vi "CVT2ParallelStaticTest.vi"() -> (3 "Unit Test Framework Results":T1)   [LabVIEW 2013, in "UnitTests.lvlib"]
uses:
  UnitTests.lvlib
  <vilib>/utf/common/utf_test_result_troll.ctl
  <vilib>/utf/common/utf_test_result.ctl
  <vilib>/utf/common/utf_test_result_failure.ctl
  <vilib>/utf/common/utf_test_comparison_operators.ctl
  <vilib>/utf/common/utf_vi_tag.ctl
  <vilib>/NI/Current Value Table/DataTypes/I32_Static Write.vi
  <vilib>/NI/Current Value Table/DataTypes/I32_Static Read.vi
  <vilib>/NI/Current Value Table/Type to Enum.vi
  <vilib>/NI/Current Value Table/DataTypes/I32_Type To Enum.vi
  <vilib>/NI/Current Value Table/FGVs/Tag Memory.vi
  <vilib>/NI/Current Value Table/Memory Block.vi
  <vilib>/NI/Current Value Table/DataTypes/I32_Memory Block.vi
  <vilib>/utf/NI_UnitTestFramework.lvlib
  <vilib>/NI/Current Value Table/Current Value Table.lvlib
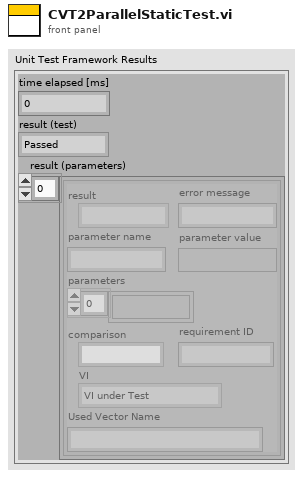
[diagram p1: front panel]
types:
  T1 = typedef "NI_UnitTestFramework.lvlib/utf_test_result_troll.ctl" = cluster{"time elapsed [ms]":u32, "result (test)":T2, "result (parameters)":T3[]}
  T2 = typedef "NI_UnitTestFramework.lvlib/utf_test_result.ctl" = enum16{"Passed", "Failed", "Error", "Skipped", "Not Processed"}
  T3 = typedef "NI_UnitTestFramework.lvlib/utf_test_result_failure.ctl" = cluster{"result":T2, "error message":string, "parameter name":string, "parameter value":variant, "parameters":variant[], "comparison":T4, "requirement ID":string, "VI":T5, "Used Vector Name":string}
  T4 = typedef "NI_UnitTestFramework.lvlib/utf_test_comparison_operators.ctl" = enum16{"=", "!=", ">", ">=", "<", "<=", "range", "symmetric tolerance", "asymmetric tolerance", "string contains", "string not contain", "array size", "string length", "array range", "by element", "array range (limit array)", "user-defined", "array contains", "array not contain", "vector length", "= (elm)", "!= (elm)", "= (case insensitive)", "!= (case insensitive)"}
  T5 = typedef "NI_UnitTestFramework.lvlib/utf_vi_tag.ctl" = enum16{"Setup VI", "VI under Test", "Teardown VI"}
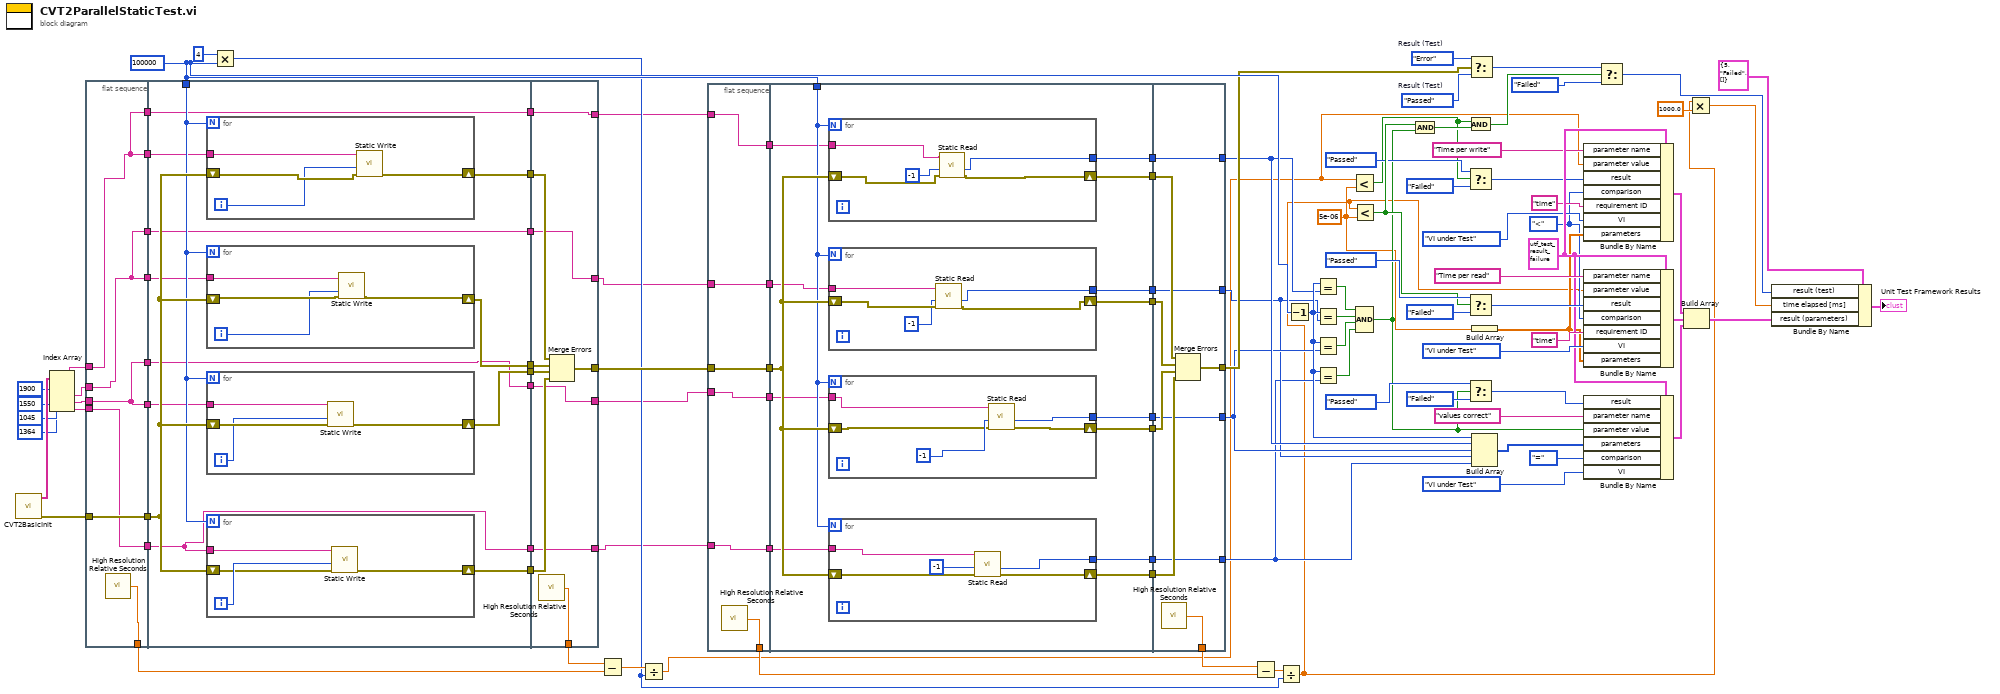
[diagram p0: block diagram]
diagram:
  w51 = T3 {"result"=enum."Passed", "error message"="", "parameter name"="", "parameter value"=variant, "parameters"=[], "comparison"=enum."=", "requirement ID"="", "VI"=enum."Setup VI", "Used Vector Name"=""} ("Unit Test Framework - result (parameters)")
  w31 = 5e-06 ("y")
  w42 = utf_test_comparison_operators."<" ("comparison")
  w87 = utf_test_result."Error"  # Result (Test)
  w86 = utf_test_result."Passed"  # Result (Test)
  w58 = 100000
  n1 = call "CVT2BasicInit.vi"() -> ("error out"=w66:errorcluster, "names"=w28:string[])  [unwired: 9 in, 1 out]
  n2 = Index Array(array=w28, index #1=1900 ("index"), index #2=1550 ("index"), index #3=1045 ("index"), index #4=1364 ("index")) -> (element #1=w17:string, element #2=w18:string, element #3=w20:string, element #4=w23:string)
  n3 = flat-sequence {
    tunnel: [w111] -> w105
    tunnel: [w112] -> w104
    tunnel: w66 -> [w112]
    tunnel: w23 -> [w110]
    tunnel: [w110] -> w22
    tunnel: [w107] -> w21
    tunnel: w20 -> [w107]
    tunnel: [w108] -> w19
    tunnel: w18 -> [w108]
    tunnel: w17 -> [w109]
    tunnel: [w109] -> w16
    tunnel: [w109] -> w12
    tunnel: [w108] -> w11
    tunnel: [w107] -> w4
    tunnel: w104 -> [w125]
    tunnel: [w124] -> w101
    tunnel: [w123] -> w100
    tunnel: [w122] -> w99
    tunnel: [w121] -> w98
    tunnel: w58 -> [w120]
    tunnel: w22 -> [w113]
    tunnel: w21 -> [w119]
    tunnel: w19 -> [w118]
    tunnel: w16 -> [w117]
    tunnel: [w116] -> w13
    tunnel: w12 -> [w116]
    tunnel: w11 -> [w115]
    tunnel: [w115] -> w10
    tunnel: [w114] -> w5
    tunnel: w4 -> [w114]
    tunnel: [w113] -> w3
    tunnel: [w146] -> w106
    tunnel: w101 -> [w151]
    tunnel: w100 -> [w150]
    tunnel: w99 -> [w149]
    tunnel: w98 -> [w148]
    tunnel: [w147] -> w92
    tunnel: [w145] -> w14
    tunnel: w13 -> [w145]
    tunnel: w10 -> [w144]
    tunnel: [w144] -> w9
    tunnel: [w143] -> w6
    tunnel: w5 -> [w143]
    tunnel: w3 -> [w142]
    tunnel: [w142] -> w2
    frame #0 {
      n4 = call <vilib>:"High Resolution Relative Seconds.vi"() -> ("relative seconds"=w111:dbl)
    }
    frame #1 {
      n5 = for {
        N: w120 -> [_]
        shift-right: [w139] -> w124
        shift-left: w125 -> [w140]
        tunnel: w117 -> [w141]
        i -> [w138]
        n6 = call-poly <vilib>:"Static Write.vi"("error in (no error)"=w140, "Value"=w138, "Tag Name"=w141) -> ("error out"=w139:errorcluster)  [unwired: 8 in]
      }
      n7 = for {
        N: w120 -> [_]
        shift-right: [w128] -> w123
        shift-left: w125 -> [w129]
        tunnel: w118 -> [w126]
        i -> [w127]
        n8 = call-poly <vilib>:"Static Write.vi"("error in (no error)"=w129, "Value"=w127, "Tag Name"=w126) -> ("error out"=w128:errorcluster)  [unwired: 8 in]
      }
      n9 = for {
        N: w120 -> [_]
        shift-right: [w137] -> w122
        shift-left: w125 -> [w136]
        tunnel: w119 -> [w134]
        i -> [w135]
        n10 = call-poly <vilib>:"Static Write.vi"("error in (no error)"=w136, "Value"=w135, "Tag Name"=w134) -> ("error out"=w137:errorcluster)  [unwired: 8 in]
      }
      n11 = for {
        N: w120 -> [_]
        shift-right: [w130] -> w121
        shift-left: w125 -> [w131]
        tunnel: w113 -> [w133]
        i -> [w132]
        n12 = call-poly <vilib>:"Static Write.vi"("error in (no error)"=w131, "Value"=w132, "Tag Name"=w133) -> ("error out"=w130:errorcluster)  [unwired: 8 in]
      }
    }
    frame #2 {
      n13 = call <vilib>:"High Resolution Relative Seconds.vi"() -> ("relative seconds"=w146:dbl)
      n14 = Merge Errors(w151, w150, w149, w148) -> (w147:errorcluster)
    }
  }
  n15 = Multiply(x=4, y=w58) -> (x*y=w54:i32)
  n16 = Subtract(x=w106, y=w105) -> (x-y=w56:dbl)
  n17 = Divide(x=w56, y=w54) -> (x/y=w29:dbl)
  n18 = flat-sequence {
    tunnel: [w156] -> w103
    tunnel: [w157] -> w97
    tunnel: w92 -> [w157]
    tunnel: [w155] -> w15
    tunnel: w14 -> [w155]
    tunnel: w9 -> [w154]
    tunnel: [w154] -> w8
    tunnel: [w153] -> w7
    tunnel: w6 -> [w153]
    tunnel: w2 -> [w152]
    tunnel: [w152] -> w1
    tunnel: w97 -> [w171]
    tunnel: [w170] -> w96
    tunnel: [w169] -> w95
    tunnel: [w168] -> w94
    tunnel: [w167] -> w93
    tunnel: w58 -> [w166]
    tunnel: [w165] -> w91
    tunnel: [w164] -> w65
    tunnel: [w163] -> w64
    tunnel: [w162] -> w63
    tunnel: w15 -> [w161]
    tunnel: w8 -> [w160]
    tunnel: w7 -> [w159]
    tunnel: w1 -> [w158]
    tunnel: [w201] -> w102
    tunnel: w96 -> [w195]
    tunnel: w95 -> [w194]
    tunnel: w94 -> [w193]
    tunnel: w93 -> [w192]
    tunnel: w91 -> [w199]
    tunnel: w65 -> [w197]
    tunnel: w64 -> [w198]
    tunnel: w63 -> [w200]
    tunnel: [w196] -> w53
    tunnel: [w195] -> w35
    tunnel: [w194] -> w33
    tunnel: [w193] -> w34
    tunnel: [w192] -> w32
    frame #0 {
      n19 = call <vilib>:"High Resolution Relative Seconds.vi"() -> ("relative seconds"=w156:dbl)
    }
    frame #1 {
      n20 = for {
        N: w166 -> [_]
        shift-right: [w191] -> w163
        shift-left: w171 -> [w187]
        tunnel: [w190] -> w170
        tunnel: w161 -> [w189]
        n21 = call-poly <vilib>:"Static Read.vi"("error in (no error)"=w187, "Default"=-1, "Tag Name"=w189) -> ("error out"=w191:errorcluster, "Value"=w190:i32)  [unwired: 7 in]
      }
      n22 = for {
        N: w166 -> [_]
        shift-right: [w172] -> w164
        shift-left: w171 -> [w175]
        tunnel: [w173] -> w169
        tunnel: w160 -> [w176]
        n23 = call-poly <vilib>:"Static Read.vi"("error in (no error)"=w175, "Default"=-1, "Tag Name"=w176) -> ("error out"=w172:errorcluster, "Value"=w173:i32)  [unwired: 7 in]
      }
      n24 = for {
        N: w166 -> [_]
        shift-right: [w183] -> w165
        shift-left: w171 -> [w184]
        tunnel: [w186] -> w168
        tunnel: w159 -> [w182]
        n25 = call-poly <vilib>:"Static Read.vi"("error in (no error)"=w184, "Default"=-1, "Tag Name"=w182) -> ("error out"=w183:errorcluster, "Value"=w186:i32)  [unwired: 7 in]
      }
      n26 = for {
        N: w166 -> [_]
        shift-right: [w177] -> w162
        shift-left: w171 -> [w181]
        tunnel: [w178] -> w167
        tunnel: w158 -> [w179]
        n27 = call-poly <vilib>:"Static Read.vi"("error in (no error)"=w181, "Default"=-1, "Tag Name"=w179) -> ("error out"=w177:errorcluster, "Value"=w178:i32)  [unwired: 7 in]
      }
    }
    frame #2 {
      n28 = call <vilib>:"High Resolution Relative Seconds.vi"() -> ("relative seconds"=w201:dbl)
      n29 = Merge Errors(w198, w197, w199, w200) -> (w196:errorcluster)
    }
  }
  n30 = Subtract(x=w102, y=w103) -> (x-y=w55:dbl)
  n31 = Divide(x=w55, y=w54) -> (x/y=w30:dbl)
  n32 = Decrement(x=w58) -> (x-1=w36:i32)
  n33 = Equal?(x=w36, y=w35) -> (x = y?=w59:bool)
  n34 = Equal?(x=w36, y=w33) -> (x = y?=w60:bool)
  n35 = Equal?(x=w36, y=w34) -> (x = y?=w61:bool)
  n36 = Equal?(x=w36, y=w32) -> (x = y?=w62:bool)
  n37 = Less?(x=w29, y=w31) -> (x < y?=w38:bool)
  n38 = Less?(x=w30, y=w31) -> (x < y?=w74:bool)
  n39 = Compound Arithmetic op=AND(w59, w60, w61, w62) -> (w37:bool)
  n40 = And(x=w74, y=w37) -> (x .and. y?=w47:bool)
  n41 = And(x=w38, y=w47) -> (x .and. y?=w46:bool)
  n42 = Select(t=utf_test_result."Passed" ("result"), s=w38, f=utf_test_result."Failed" ("result")) -> (s? t:f=w39:T2)
  n43 = Select(t=utf_test_result."Passed" ("result"), s=w74, f=utf_test_result."Failed" ("result")) -> (s? t:f=w77:T2)
  n44 = Select(t=utf_test_result."Passed" ("result"), s=w37, f=utf_test_result."Failed" ("result")) -> (s? t:f=w70:T2)
  n45 = Select(t=w87, s=w53, f=w86) -> (s? t:f=w82:T2)
  n46 = Build Array(w31) -> (w43:dbl[])
  n47 = Build Array(w36, w35, w34, w33, w32) -> (w68:i32[])
  n48 = Bundle By Name(cluster=w51, "parameter name"="Time per write", "parameter value"=w29, "result"=w39, "comparison"=w42, "requirement ID"="time", "VI"=utf_vi_tag."VI under Test", "parameters"=w43) -> (w52:T3)
  n49 = Bundle By Name(cluster=w51, "parameter name"="Time per read", "parameter value"=w30, "result"=w77, "comparison"=w42, "requirement ID"="time", "VI"=utf_vi_tag."VI under Test", "parameters"=w43) -> (w50:T3)
  n50 = Bundle By Name(cluster=w51, "result"=w70, "parameter name"="values correct", "parameter value"=w37, "parameters"=w68, "comparison"=utf_test_comparison_operators."=", "VI"=utf_vi_tag."VI under Test") -> (w49:T3)
  n51 = Select(t=w82, s=w46, f=utf_test_result."Failed") -> (s? t:f=w80:T2)
  n52 = Build Array(w52, w50, w49) -> (w85:T3[])
  n53 = Multiply(x=w30, y=1000.0) -> (x*y=w83:dbl)
  n54 = Bundle By Name(cluster=T1 {"time elapsed [ms]"=5, "result (test)"=enum."Failed", "result (parameters)"=[]} ("Unit Test Framework - Result"), "result (test)"=w80, "time elapsed [ms]"=w83, "result (parameters)"=w85) -> (→"Unit Test Framework Results":T1)
